vi "Agilent SNA Compute Timeout.vi"(5 "Points":dbl, 7 "IFBW (Hz)":dbl, 9 "Sweep Time (s)":dbl) -> (8 "Timeout (ms)":dbl)   [LabVIEW 2011]
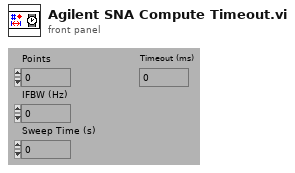
[diagram p1: front panel]
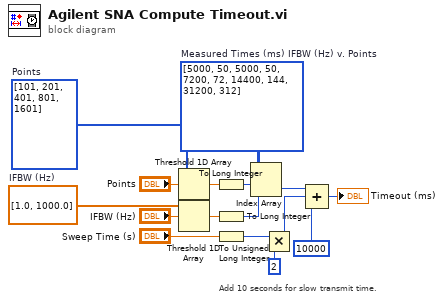
[diagram p0: block diagram]
diagram:
  w8 = dbl[] [1.0, 1000.0]  # IFBW (Hz)
  w9 = i32[] [101, 201, 401, 801, 1601]  # Points
  w16 = u32[][] [[5000, 50], [5000, 50], [7200, 72], [14400, 144], [31200, 312]]  # Measured Times (ms) IFBW (Hz) v. Points
  # "Add 10 seconds for slow transmit time."
  n1 = Threshold 1D Array(2:"Points", 3:w9) -> (0:w15:dbl)  [unwired: 1 out]
  n2 = Threshold 1D Array(2:"IFBW (Hz)", 3:w8) -> (0:w12:dbl)  [unwired: 1 out]
  n3 = To Long Integer(number=w15) -> (32bit integer=w13:i32)
  n4 = To Long Integer(number=w12) -> (32bit integer=w11:i32)
  n5 = To Unsigned Long Integer(number="Sweep Time (s)") -> (unsigned 32bit integer=w2:u32)
  n6 = Index Array(array=w16, index (row)=w13, index (col)=w11) -> (element=w6:u32)
  n7 = Multiply(x=w2, y=2) -> (x*y=w1:u32)
  n8 = Compound Arithmetic op=ADD(w6, w1, u32 10000 ("y")) -> (→"Timeout (ms)":u32)
